vi "Read Msg.vi"(11 "Base Actor in":refnum<class "Base Actor.lvclass">) -> (2 "Msg":refnum<class "Msg.lvclass">)   [LabVIEW 2025, in "jettl.lvlib" / "Base jettl Actor.lvlib" / "Base Actor.lvlib" / "Base Actor.lvclass"]
uses:
  Base Actor.lvclass
  Msg/Msg.lvclass
  Base Actor.lvclass/Base Actor.ctl
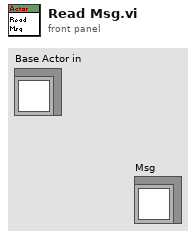
[diagram p1: front panel]
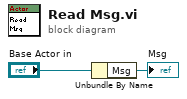
[diagram p0: block diagram]
diagram:
  n1 = Unbundle By Name("Base Actor in") -> ("Msg"=→"Msg":refnum<class "Msg.lvclass">)
